vi "HFRR ADV v037 new software.vi"() -> ()   [LabVIEW 2025] (continued)
                    n909 = Number To Fractional String(number=w1103, precision (6)=i16 1) -> (F-format string=w1102:string)  [unwired: 2 in]
                    n910 = local write "Minor Axis"(w1108) -> ()
                    n911 = local write "Major Axis"(w1108) -> ()
                    n912 = Fract/Exp String To Number(string=w1102) -> (number=w1101:dbl)  [unwired: 3 in, 1 out]
                    n913 = local write "Average"(w1101) -> ()
                  }
                }
              }
              frame True {
                w1140 = 1000.0 ("y")
                w1146 = 0.0 ("default (0 DBL)")
                n914 = Match Pattern(string=w1152, regular expression=" \"width_px\":") -> (after substring=w1150:string)  [unwired: 1 in, 3 out]
                n915 = Match Pattern(string=w1150, regular expression="\"height_px\":") -> (before substring=w1148:string, after substring=w1147:string)  [unwired: 1 in, 2 out]
                n916 = Fract/Exp String To Number(string=w1148, default (0 dbl)=w1146) -> (number=w1145:dbl)  [unwired: 2 in, 1 out]
                n917 = Fract/Exp String To Number(string=w1147, default (0 dbl)=w1146) -> (number=w1144:dbl)  [unwired: 2 in, 1 out]
                n918 = Multiply(x=w1145, y=w1143) -> (x*y=w1142:dbl)
                n919 = Multiply(x=w1144, y=w1143) -> (x*y=w1141:dbl)
                n920 = Multiply(x=w1142, y=w1140) -> (x*y=w1126:dbl)
                n921 = Multiply(x=w1141, y=w1140) -> (x*y=w1124:dbl)
                n922 = Add(x=w1126, y=w1124) -> (x+y=w1138:dbl)
                n923 = property on="Major Axis" class="DigNum (strict)"("Caption.Text"="Major Axis") -> ()  [unwired: 2 in, 2 out]
                n924 = property on="Minor Axis" class="DigNum (strict)"("Caption.Text"="Minor Axis") -> ()  [unwired: 2 in, 2 out]
                n925 = property on="Average" class="DigNum (strict)"("Caption.Text"="Average") -> ()  [unwired: 2 in, 2 out]
                n926 = Divide(x=w1138, y=2.0) -> (x/y=w1122:dbl)
                n927 = Bundle By Name(cluster=w1139, "major"=w1126, "minor"=w1124, "average"=w1122) -> (w1136:cluster{"major":dbl, "minor":dbl, "average":dbl})
                n928 = Number To Fractional String(number=w1124, precision (6)=i16 1) -> (F-format string=w1131:string)  [unwired: 2 in]
                n929 = Number To Fractional String(number=w1122, precision (6)=i16 1) -> (F-format string=w1132:string)  [unwired: 2 in]
                n930 = Number To Fractional String(number=w1126, precision (6)=i16 1) -> (F-format string=w1130:string)  [unwired: 2 in]
                n931 = Fract/Exp String To Number(string=w1131) -> (number=w1123:dbl)  [unwired: 3 in, 1 out]
                n932 = Fract/Exp String To Number(string=w1132) -> (number=w1121:dbl)  [unwired: 3 in, 1 out]
                n933 = Fract/Exp String To Number(string=w1130) -> (number=w1125:dbl)  [unwired: 3 in, 1 out]
                n934 = local write "Major Axis"(w1125) -> ()
                n935 = local write "Average"(w1121) -> ()
                n936 = local write "Minor Axis"(w1123) -> ()
              }
            }
            n937 = case shown="\"Measrument\", Default" w1032 {
              tunnel: w1035 -> [w1065 _]
              tunnel: w1034 -> [w1064 _]
              tunnel: [w1061 w1090] -> w1033
              tunnel: w1031 -> [w1063 w1090]
              tunnel: w1030 -> [w1062 _]
              tunnel: w1027 -> [w1060 _]
              frame "Measrument", Default {
                n938 = stacked-sequence {
                  tunnel: w1065 -> [w1083 _]
                  tunnel: w1064 -> [w1081 _]
                  tunnel: w1063 -> [w1079 _]
                  tunnel: w1062 -> [w1078 _]
                  tunnel: [w1073 _] -> w1061
                  tunnel: w1060 -> [w1066 _]
                  frame #0 {
                    n939 = call "IMAGE ANALYSIS.vi"("Enum"=POST_ANALYSIS_ENUM."SAVE IMAGE", "error in"=w1079, "IMAGE FILE PATH"=w1078) -> ("error out"=w1077:errorcluster)  [unwired: 7 in, 1 out]
                    n940 = call "Stall Data Flow.vim"("value in"=w1077, "milliseconds to wait"=u32 1000) -> ("value out"=w1068:errorcluster)  [unwired: 1 out]
                    n941 = local read "Test File List :"() -> (w1085:string)
                    n942 = call "IMAGE ANALYSIS.vi"("Enum"=POST_ANALYSIS_ENUM."MINIMIZE UI", "error in"=w1068) -> ("error out"=w1075:errorcluster)  [unwired: 8 in, 1 out]
                    n943 = Bundle By Name(cluster=T26 {"File Name"="", "Test Method"="", "Operator"="", "Fuel Description"="", "Date and time"=""} ("Main Ref"), "Test Method"=w1066, "File Name"=w1085) -> (w1086:T26)
                    n944 = call "Stall Data Flow.vim"("value in"=w1075, "milliseconds to wait"=u32 1500) -> ("value out"=w1070:errorcluster)  [unwired: 1 out]
                    n945 = call "duf file read.vi"("error in (no error)"=w1070, "Main Ref"=w1086) -> ("error out"=w1084:errorcluster, "Main Ref 2"=w1082:T26)  [unwired: 8 in]
                    n946 = call "DETECTION REPORT for manual.vi"("error in (no error)"=w1084, "return value 3"=w1081, "Image File Path"=w1083, "Main Ref"=w1082) -> ("error out"=w1080:errorcluster)  [unwired: 7 in]
                    n947 = call <vilib>:"Clear Errors.vi"("error in (no error)"=w1080) -> ("error out"=w1071:errorcluster)  [unwired: 5 in, 1 out]
                    n948 = call "IMAGE ANALYSIS.vi"("Enum"=POST_ANALYSIS_ENUM."MINIMIZE UI", "error in"=w1071) -> ("error out"=w1073:errorcluster)  [unwired: 8 in, 1 out]
                  }
                  frame #1 {
                    n949 = local write "Main Tab"(T2."HOME" ("Main Tab")) -> ()
                    n950 = local write "Main Dashboard Buttons"(T1."Home" ("Main Dashboard Buttons")) -> ()
                  }
                }
              }
              frame "Calibrate" {
              }
            }
          }
          frame #2 {
            n951 = Not(x=w1155) -> (.not. x?=w1154:bool)
            n952 = local write "Confirm Measrurement"(w1154) -> ()
            n953 = local read "Calibration Tab"() -> (w1153:enum32{"Measrument", "Calibrate"})
            n954 = case shown="\"Measrument\", Default" w1153 {
              frame "Measrument", Default {
                (unwired) T21."HOME" ("Main Tab")
                n955 = local write "Main Tab"(T2."HOME" ("Main Tab")) -> ()
              }
              frame "Calibrate" {
              }
            }
          }
        }
      }
    }
    n956 = local read "Humidity"() -> (w889:bool)
    n957 = local read "Save Change"() -> (w894:bool)
    n958 = local read "Calibrate"() -> (w895:bool)
    n959 = local read "Auto Start Test"() -> (w890:bool)
    n960 = case shown="True" w895 {
      selector: w895 -> [_ w1002]
      frame False {
      }
      frame True {
        n961 = Not(x=w1002) -> (.not. x?=w1001:bool)
        n962 = local write "Calibrate"(w1001) -> ()
        n963 = local write "Calibration Tab"(enum32{"Measrument", "Calibrate"}."Calibrate" ("Calibration Tab")) -> ()
      }
    }
    n964 = case shown="True" w894 {
      selector: w894 -> [_ w946]
      frame False {
      }
      frame True {
        n965 = stacked-sequence {
          tunnel: w946 -> [_ _ _ _ w1000]
          frame #0 {
            n966 = call "IMAGE ANALYSIS.vi"("Enum"=POST_ANALYSIS_ENUM."HIDE UI") -> ()  [unwired: 9 in, 2 out]
          }
          frame #1 {
            n967 = local read "100x gain"() -> (w948:dbl)
            n968 = local read "10x Gain"() -> (w949:dbl)
            n969 = local read "5x Gain"() -> (w950:dbl)
            n970 = Number To Fractional String(number=w949, width (-)=i16 4, precision (6)=i16 7) -> (F-format string=w971:string)  [unwired: 1 in]
            n971 = Number To Fractional String(number=0.0, width (-)=i16 4, precision (6)=i16 7) -> (F-format string=w966:string)  [unwired: 1 in]
            n972 = Number To Fractional String(number=w948, width (-)=i16 4, precision (6)=i16 7) -> (F-format string=w954:string)  [unwired: 1 in]
            n973 = Number To Fractional String(number=w950, width (-)=i16 10 ("precision (6)"), precision (6)=i16 7) -> (F-format string=w980:string)  [unwired: 1 in]
            n974 = Concatenate Strings("[CH1]" ("string"), w980, " - 5x Gain" ("string"), "\r") -> (w970:string)
            n975 = Concatenate Strings("[CH2]" ("string"), w971, " - 10x Gain" ("string"), "\r") -> (w969:string)
            n976 = Concatenate Strings("[CH3]" ("string"), w966, " - 20x Gain" ("string"), "\r") -> (w960:string)
            n977 = Concatenate Strings("[CH4]" ("string"), w954, " - 100x Gain" ("string"), "\r") -> (w953:string)
            n978 = String To Path(string="C:\\LAB-IQ\\Image Calibrate v01.dcf") -> (path=w983:path)
            n979 = Concatenate Strings(w970, w969, w960, w953) -> (w968:string)
            n980 = call <vilib>:"Write Characters To File.vi"("append to file? (new file:F)"=FALSE, "character string"=w968, "file path (dialog if empty)"=w983) -> ()  [unwired: 2 in, 1 out]
          }
          frame #2 {
            n981 = String To Path(string="C:\\LAB-IQ\\Image Calibrate v01.dcf") -> (path=w986:path)
            n982 = Open/Create/Replace File ("Open File")(file path (use dialog)=w986) -> (refnum out=w987:refnum<file>)  [unwired: 5 in, 2 out]
            n983 = for {
              N: 4 -> [_]
              tunnel: w987 -> [w993]
              i -> [w989]
              n984 = Read from Text File ("Read File")(file (use dialog)=w993) -> (text=w994:string)  [unwired: 3 in, 3 out]
              n985 = String Subset(string=w994, offset (0)=6, length (rest)=10 ("length (rest)")) -> (substring=w990:string)
              n986 = Fract/Exp String To Number(string=w990) -> (number=w988:dbl)  [unwired: 3 in, 1 out]
              n987 = case shown="3" w989 {
                tunnel: w988 -> [w995 w996 _ w997 _]
                frame 0 {
                  n988 = local write "5x Gain"(w995) -> ()
                }
                frame 1 {
                  n989 = local write "10x Gain"(w996) -> ()
                }
                frame 2 {
                }
                frame 3 {
                  n990 = local write "100x gain"(w997) -> ()
                }
                frame 4, Default {
                }
              }
            }
          }
          frame #3 {
            n991 = call "IMAGE ANALYSIS.vi"("Enum"=POST_ANALYSIS_ENUM."SHOW UI") -> ()  [unwired: 9 in, 2 out]
          }
          frame #4 {
            n992 = Not(x=w1000) -> (.not. x?=w999:bool)
            n993 = local write "Save Change"(w999) -> ()
          }
        }
      }
    }
    n994 = case shown="False" w890 {
      tunnel: w889 -> [w916 _]
      frame False {
        n995 = case shown="True" w916 {
          frame False {
          }
          frame True {
            n996 = local read "Set Humidity:"() -> (w920:dbl)
            n997 = local read "Set Humidity:"() -> (w923:dbl)
            n998 = local read "Humidity ( %RH )"() -> (w924:dbl)
            n999 = Subtract(x=w920, y=2.0) -> (x-y=w918:dbl)
            n1000 = Add(x=w923, y=2.0) -> (x+y=w919:dbl)
            n1001 = In Range and Coerce(upper limit=w919, x=w924, lower limit=w918) -> (In Range?=w917:bool)  [unwired: 1 out]
            n1002 = case shown="True" w917 {
              frame False {
              }
              frame True {
                n1003 = case shown="True" "Manual Humididty Reached" {
                  selector: "Manual Humididty Reached" -> [_ w927]
                  frame False {
                  }
                  frame True {
                    n1004 = Not(x=w927) -> (.not. x?=w926:bool)
                    n1005 = local write "Manual Humididty Reached"(w926) -> ()
                    n1006 = local read "EVENT LOG"() -> (w929:string)
                    n1007 = call "Event Log.vi"("Content"="Target Humidity reached", "EVENT LOG"=w929) -> ("EVENT LOG"=w928:string)  [unwired: 8 in, 1 out]
                    n1008 = local write "EVENT LOG"(w928) -> ()
                  }
                }
              }
            }
          }
        }
      }
      frame True {
        n1009 = local write "Manual Humididty Reached"(TRUE ("Manual Humididty Reached")) -> ()
      }
    }
    n1010 = Wait (ms)(milliseconds to wait=u32 250) -> ()  [unwired: 1 out]
    n1011 = local read "Cap Live Image"() -> (w910:bool)
    n1012 = local read "SCAR MEASURMENT"() -> (w913:enum32{"Auto Scar", "Manual Scar"})
    n1013 = Equal?(x=w913, y=enum32{"Auto Scar", "Manual Scar"}."Manual Scar" ("SCAR MEASURMENT")) -> (x = y?=w911:bool)
    n1014 = And(x=w911, y=w910) -> (x .and. y?=w909:bool)
    n1015 = case shown="True" w909 {
      selector: w909 -> [_ w1241]
      frame False {
      }
      frame True {
        n1016 = stacked-sequence {
          tunnel: [_ _ _ w1260 _] -> _
          tunnel: w1241 -> [_ _ _ _ w1267]
          frame #0 {
            w1242 = 0.0
            n1017 = local write "Major Axis"(w1242) -> ()
            n1018 = local write "Minor Axis"(w1242) -> ()
            n1019 = local write "Average"(w1242) -> ()
          }
          frame #1 {
            n1020 = call "CAMERA LIVE FEED FGV.vi"("Enum - Menu"=CAMERA_LIVE_FEED_ENUM."CAMERA MINIMIZE") -> ()  [unwired: 9 in, 2 out]
          }
          frame #2 {
            n1021 = local read "Magnification len live scar"() -> (w1245:string)
            n1022 = case shown="\"10x\", Default" w1245 {
              tunnel: ["_10x" "_5x"] -> w1244
              frame "10x", Default {
              }
              frame "5x" {
              }
            }
            n1023 = local read "FILE 3"() -> (w1252:string)
            n1024 = call <vilib>:"Trim Whitespace.vi"("string"="C:\\LAB-IQ\\images\\") -> ("trimmed string"=w1254:string)  [unwired: 1 in]
            n1025 = String To Path(string=w1254) -> (path=w1253:path)
            n1026 = Concatenate Strings(w1252, w1244, ".png" ("string")) -> (w1251:string)
            n1027 = Build Path(base path=w1253, name or relative path=w1251) -> (appended path=w1250:path)
            n1028 = Path To String(path=w1250) -> (string=w1249:string)
            n1029 = call "CAMERA LIVE FEED FGV.vi"("Enum - Menu"=CAMERA_LIVE_FEED_ENUM."CAMERA SAVE", "Image Path"=w1249) -> ("error out"=w1247:errorcluster)  [unwired: 8 in, 1 out]
            n1030 = case shown="No Error" w1247 {
              frame No Error {
                n1031 = One Button Dialog(message="Image saved successfully") -> ()  [unwired: 1 in, 1 out]
              }
              frame Error {
              }
            }
          }
          frame #3 {
            n1032 = call "LIST FILE NAMES.vi"() -> ("error out"=w1262:errorcluster, "filenames"=w1259:string[])  [unwired: 10 in]
            n1033 = call "IMAGE ANALYSIS.vi"("Enum"=POST_ANALYSIS_ENUM."SHOW UI", "error in"=w1262) -> ("error out"=w1260:errorcluster)  [unwired: 8 in, 1 out]
            n1034 = property on="Test File List :" class="CmbBox"("Strings[]"=w1259) -> ()  [unwired: 2 in, 2 out]
          }
          frame #4 {
            (unwired) T25."Report" ("Main Dashboard Buttons")
            (unwired) T27."Report" ("Main Dashboard Buttons")
            n1035 = Not(x=w1267) -> (.not. x?=w1266:bool)
            n1036 = local write "Zoom Factore"(0.0 ("Zoom Factore")) -> ()
            n1037 = local write "Cap Live Image"(w1266) -> ()
            n1038 = local write "Main Tab"(T2."Adv Scar Report" ("Main Tab")) -> ()
            n1039 = property on="Cap Live Image" class="Bool (strict)"("BoolText.Text"="Capture Image" ("Boolean Text.Text")) -> ()  [unwired: 2 in, 2 out]
            n1040 = local write "Main Dashboard Buttons"(T1."Report" ("Main Dashboard Buttons")) -> ()
          }
        }
      }
    }
    n1041 = local read "change Gain"() -> (w893:bool)
    n1042 = local read "Back Square"() -> (w892:bool)
    n1043 = case shown="True" w893 {
      selector: w893 -> [_ w937]
      frame False {
      }
      frame True {
        n1044 = stacked-sequence {
          tunnel: w937 -> [_ w945]
          frame #0 {
            n1045 = local read "Actual (µm)"() -> (w941:dbl)
            n1046 = local read "Pixel Value"() -> (w940:dbl)
            n1047 = local read "Magnification :"() -> (w939:string)
            n1048 = Divide(x=w941, y=w940) -> (x/y=w938:dbl)
            n1049 = case shown="\"10x\"" w939 {
              tunnel: w938 -> [w942 w943]
              frame "10x" {
                n1050 = local write "10x Gain"(w942) -> ()
              }
              frame "5x", Default {
                n1051 = local write "5x Gain"(w943) -> ()
              }
            }
          }
          frame #1 {
            n1052 = Not(x=w945) -> (.not. x?=w944:bool)
            n1053 = local write "change Gain"(w944) -> ()
          }
        }
      }
    }
    n1054 = case shown="True" w892 {
      selector: w892 -> [_ w935]
      frame False {
      }
      frame True {
        n1055 = Not(x=w935) -> (.not. x?=w934:bool)
        n1056 = local write "Back Square"(w934) -> ()
        n1057 = local write "Calibration Tab"(enum32{"Measrument", "Calibrate"}."Measrument" ("Calibration Tab")) -> ()
      }
    }
    n1058 = local read "Rectangle Tool"() -> (w904:bool)
    n1059 = local read "Clear ROI Tool"() -> (w903:bool)
    n1060 = local read "Open Image"() -> (w908:bool)
    n1061 = local read "line tool"() -> (w905:bool)
    n1062 = local read "OUT"() -> (w906:bool)
    n1063 = local read "In"() -> (w907:bool)
    n1064 = case shown="True" w908 {
      selector: w908 -> [_ w1227]
      tunnel: [w1218 w1229] -> _
      tunnel: w898 -> [w1218 w1228]
      frame False {
      }
      frame True {
        w1220 = "_5x" ("regular expression")
        n1065 = Not(x=w1227) -> (.not. x?=w1226:bool)
        n1066 = local write "Open Image"(w1226) -> ()
        n1067 = call "IMAGE ANALYSIS.vi"("Enum"=POST_ANALYSIS_ENUM."HIDE UI", "error in"=w1228) -> ("error out"=w1236:errorcluster)  [unwired: 8 in, 1 out]
        n1068 = call "File Dialog"("start path"=path "C:/LAB-IQ/images", "error in"=w1236) -> ("selected path"=w1225:path, "error out"=w1234:errorcluster)  [unwired: 10 in, 2 out]
        "Image path  2" <- w1225
        n1069 = call <vilib>:"Clear Errors.vi"("error in (no error)"=w1234) -> ("error out"=w1233:errorcluster)  [unwired: 5 in, 1 out]
        n1070 = call "IMAGE ANALYSIS.vi"("Enum"=POST_ANALYSIS_ENUM."OPEN FILE", "error in"=w1233, "File Path"=w1225) -> ("error out"=w1232:errorcluster)  [unwired: 7 in, 1 out]
        n1071 = call <vilib>:"Clear Errors.vi"("error in (no error)"=w1232) -> ("error out"=w1231:errorcluster)  [unwired: 5 in, 1 out]
        n1072 = call "IMAGE ANALYSIS.vi"("Enum"=POST_ANALYSIS_ENUM."SHOW UI", "error in"=w1231) -> ("error out"=w1229:errorcluster)  [unwired: 8 in, 1 out]
        n1073 = local write "Zoom Factore"(100.0 ("Zoom Factore")) -> ()
        n1074 = local read "Image path  2"() -> (w1221:path)
        n1075 = Strip Path(path=w1221) -> (name=w1223:string)  [unwired: 1 out]
        n1076 = Match Pattern(string=w1223, regular expression=w1220) -> (match substring=w1222:string)  [unwired: 1 in, 3 out]
        n1077 = Equal?(x=w1222, y=w1220) -> (x = y?=w1219:bool)
        n1078 = case shown="True" w1219 {
          frame False {
            n1079 = local write "Magnification :"("10x" ("Magnification :")) -> ()
          }
          frame True {
            n1080 = local write "Magnification :"("5x" ("Magnification :")) -> ()
          }
        }
      }
    }
    n1081 = case shown="True" w906 {
      selector: w906 -> [_ w1203]
      tunnel: w898 -> [w1200 w1208]
      tunnel: [w1200 w1202] -> _
      frame False {
      }
      frame True {
        n1082 = Not(x=w1203) -> (.not. x?=w1201:bool)
        n1083 = local read "Zoom Factore"() -> (w1206:dbl)
        n1084 = local write "OUT"(w1201) -> ()
        n1085 = call "IMAGE ANALYSIS.vi"("Enum"=POST_ANALYSIS_ENUM."ZOOM OUT", "error in"=w1208) -> ("error out"=w1202:errorcluster)  [unwired: 8 in, 1 out]
        n1086 = Divide(x=w1206, y=1.2) -> (x/y=w1204:dbl)
        n1087 = local write "Zoom Factore"(w1204) -> ()
      }
    }
    n1088 = case shown="True" w907 {
      selector: w907 -> [_ w1212]
      tunnel: w898 -> [w1209 w1217]
      tunnel: [w1209 w1210] -> _
      frame False {
      }
      frame True {
        n1089 = Not(x=w1212) -> (.not. x?=w1211:bool)
        n1090 = local read "Zoom Factore"() -> (w1215:dbl)
        n1091 = local write "In"(w1211) -> ()
        n1092 = call "IMAGE ANALYSIS.vi"("Enum"=POST_ANALYSIS_ENUM."ZOOM IN", "error in"=w1217) -> ("error out"=w1210:errorcluster)  [unwired: 8 in, 1 out]
        n1093 = Multiply(x=w1215, y=1.2) -> (x*y=w1213:dbl)
        n1094 = local write "Zoom Factore"(w1213) -> ()
      }
    }
    n1095 = case shown="True" w903 {
      selector: w903 -> [_ w1184]
      tunnel: w898 -> [w1182 w1186]
      tunnel: [w1182 w1185] -> _
      frame False {
      }
      frame True {
        n1096 = Not(x=w1184) -> (.not. x?=w1183:bool)
        n1097 = local write "Clear ROI Tool"(w1183) -> ()
        n1098 = call "IMAGE ANALYSIS.vi"("Enum"=POST_ANALYSIS_ENUM."CLEAR ROI", "error in"=w1186) -> ("error out"=w1185:errorcluster)  [unwired: 8 in, 1 out]
      }
    }
    n1099 = case shown="True" w905 {
      selector: w905 -> [_ w1196]
      tunnel: w898 -> [w1194 w1199]
      tunnel: [w1194 w1197] -> _
      frame False {
      }
      frame True {
        n1100 = Not(x=w1196) -> (.not. x?=w1195:bool)
        n1101 = local write "line tool"(w1195) -> ()
        n1102 = call "IMAGE ANALYSIS.vi"("Enum"=POST_ANALYSIS_ENUM."DRAW LINE", "error in"=w1199) -> ("error out"=w1197:errorcluster)  [unwired: 8 in, 1 out]
      }
    }
    n1103 = case shown="True" w904 {
      selector: w904 -> [_ w1190]
      tunnel: w898 -> [w1188 w1192]
      tunnel: [w1188 w1191] -> _
      frame False {
      }
      frame True {
        n1104 = Not(x=w1190) -> (.not. x?=w1189:bool)
        n1105 = local write "Rectangle Tool"(w1189) -> ()
        n1106 = call "IMAGE ANALYSIS.vi"("Enum"=POST_ANALYSIS_ENUM."DRAW REC", "error in"=w1192) -> ("error out"=w1191:errorcluster)  [unwired: 8 in, 1 out]
      }
    }
    n1107 = local read "SCAR MEASURMENT"() -> (w891:enum32{"Auto Scar", "Manual Scar"})
    n1108 = local read "Fit to Screen Tool"() -> (w900:bool)
    n1109 = local read "Resize Tool"() -> (w899:bool)
    n1110 = case shown="\"Manual Scar\", Default" w891 {
      frame "Auto Scar" {
        n1111 = property on="Cap Live Image" class="Bool (strict)"("BoolText.Text"="Report" ("Boolean Text.Text")) -> ()  [unwired: 2 in, 2 out]
      }
      frame "Manual Scar", Default {
        n1112 = property on="Cap Live Image" class="Bool (strict)"("BoolText.Text"="Save Image" ("Boolean Text.Text")) -> ()  [unwired: 2 in, 2 out]
      }
    }
    n1113 = local read "ROI Color Tool"() -> (w901:bool)
    n1114 = local read "Pan Tool"() -> (w902:bool)
    n1115 = case shown="True" w902 {
      selector: w902 -> [_ w1178]
      tunnel: w898 -> [w1176 w1180]
      tunnel: [w1176 w1179] -> _
      frame False {
      }
      frame True {
        n1116 = Not(x=w1178) -> (.not. x?=w1177:bool)
        n1117 = call "IMAGE ANALYSIS.vi"("Enum"=POST_ANALYSIS_ENUM."PAN", "error in"=w1180) -> ("error out"=w1179:errorcluster)  [unwired: 8 in, 1 out]
        n1118 = local write "Pan Tool"(w1177) -> ()
      }
    }
    n1119 = case shown="True" w899 {
      selector: w899 -> [_ w1162]
      tunnel: w898 -> [w1157 w1159]
      tunnel: [w1157 w1158] -> _
      frame False {
      }
      frame True {
        n1120 = Not(x=w1162) -> (.not. x?=w1161:bool)
        n1121 = local write "Resize Tool"(w1161) -> ()
        n1122 = call "IMAGE ANALYSIS.vi"("Enum"=POST_ANALYSIS_ENUM."RESIZE MODE", "error in"=w1159) -> ("error out"=w1158:errorcluster)  [unwired: 8 in, 1 out]
      }
    }
    n1123 = case shown="True" w900 {
      selector: w900 -> [_ w1167]
      tunnel: [w1163 w1168] -> _
      tunnel: w898 -> [w1163 w1166]
      frame False {
      }
      frame True {
        n1124 = Not(x=w1167) -> (.not. x?=w1165:bool)
        n1125 = local write "Zoom Factore"(100.0 ("Zoom Factore")) -> ()
        n1126 = local write "Fit to Screen Tool"(w1165) -> ()
        n1127 = call "IMAGE ANALYSIS.vi"("Enum"=POST_ANALYSIS_ENUM."FIT", "error in"=w1166) -> ("error out"=w1168:errorcluster)  [unwired: 8 in, 1 out]
      }
    }
    n1128 = case shown="True" w901 {
      selector: w901 -> [_ w1173]
      tunnel: [w1170 w1174] -> _
      tunnel: w898 -> [w1170 w1171]
      frame False {
      }
      frame True {
        n1129 = Not(x=w1173) -> (.not. x?=w1172:bool)
        n1130 = local write "ROI Color Tool"(w1172) -> ()
        n1131 = call "IMAGE ANALYSIS.vi"("Enum"=POST_ANALYSIS_ENUM."SET ROI COLOR", "error in"=w1171) -> ("error out"=w1174:errorcluster)  [unwired: 8 in, 1 out]
      }
    }
    n1132 = local read "Quit"() -> (w915:bool)
  }
  n1133 = while {
    stop <- w1269 stop-if-true
    n1134 = local read "Image Path"() -> (w1272:path)
    n1135 = local read "Print 3"() -> (w1275:bool)
    n1136 = Equal?(x=w1272, y=path "") -> (x = y?=w1271:bool)
    n1137 = Not(x=w1271) -> (.not. x?=w1270:bool)
    n1138 = property on="Print 3" class="Bool (strict)"("Visible"=w1270) -> ()  [unwired: 2 in, 2 out]
    n1139 = case shown="True" w1275 {
      frame False {
        n1140 = local write "Rd"(TRUE ("Boolean 7")) -> ()
      }
      frame True {
        n1141 = flat-sequence {
          tunnel: [w1315] -> w1283
          tunnel: [w1302] -> w1281
          tunnel: [w1312] -> w1277
          tunnel: w1283 -> [w1324]
          tunnel: [w1324] -> w1282
          tunnel: w1281 -> [w1323]
          tunnel: [w1323] -> w1280
          tunnel: [w1321] -> w1279
          tunnel: [w1320] -> w1278
          tunnel: w1277 -> [w1320]
          tunnel: w1282 -> [w1326]
          tunnel: w1280 -> [w1327]
          tunnel: w1279 -> [_]
          tunnel: w1278 -> [w1325]
          frame #0 {
            n1142 = case shown="True" "Rd" {
              frame False {
              }
              frame True {
                n1143 = while {
                  tunnel: "abcdefABCDEF" ("string 2") -> [w1294]
                  shift-right: [w1292] -> w1286
                  shift-left: "" -> [w1291]
                  i -> [w1301]
                  stop <- w1300 stop-if-true
                  n1144 = Random Number (0-1)() -> (number: 0 to 1=w1295:dbl)
                  n1145 = Multiply(x=w1295, y=62.0) -> (x*y=w1297:dbl)
                  n1146 = Decrement(x="Length 2") -> (x-1=w1290:i16)
                  n1147 = To Word Integer(number=w1297) -> (16bit integer=w1298:i16)
                  n1148 = String Subset(string=w1294, offset (0)=w1298, length (rest)=1 ("length (rest)")) -> (substring=w1293:string)
                  n1149 = Greater Or Equal?(x=w1301, y=w1290) -> (x >= y?=w1300:bool)
                  n1150 = Concatenate Strings(w1293, w1291) -> (w1292:string)
                }
                "String 10" <- w1286
                n1151 = local write "Rd"(FALSE ("Boolean 7")) -> ()
              }
            }
          }
          frame #1 {
            w1313 = "_resized.jpg" ("command line")
            (unwired) ".jpg -resize 320x240 " ("string")
            (unwired) "Choose an Image File" ("prompt")
            # "-resize 1798x425"
            n1152 = local read "Image Path"() -> (w1307:path)
            n1153 = Strip Path(path=w1307) -> (stripped path=w1302:path, name=w1303:string)
            n1154 = Match Pattern(string=w1303, regular expression=".jpg") -> (before substring=→"before substring 2":string, after substring=→"after substring":string)  [unwired: 1 in, 2 out]
            n1155 = Match Pattern(string=w1303, regular expression="\\") -> (before substring=w1309:string)  [unwired: 1 in, 3 out]
            n1156 = Match Pattern(string=w1309, regular expression=".jpg") -> (before substring=w1308:string)  [unwired: 1 in, 3 out]
            n1157 = Concatenate Strings("cmd /c convert " ("string"), w1308, ".jpg -resize 320x240  " ("command line"), w1308, w1313) -> (w1316:string)
            n1158 = call <vilib>:"System Exec.vi"("run minimized? (F)"=TRUE, "wait until completion? (T)"=TRUE, "working directory"=w1302, "command line"=w1316) -> ("error out"=w1315:errorcluster)  [unwired: 4 in, 3 out]
            "error out 2" <- w1315
            n1159 = Concatenate Strings(w1308, w1313) -> (w1312:string)
          }
          frame #2 {
            n1160 = Wait (ms)(milliseconds to wait=u32 2000 ("millisecond timer value")) -> (millisecond timer value=w1321:u32)
          }
          frame #3 {
            n1161 = case shown="No Error" w1326 {
              tunnel: w1327 -> [w1330 _]
              tunnel: w1325 -> [w1328 _]
              frame No Error {
                (unwired) ".jpg" ("string")
                n1162 = Path To String(path=w1330) -> (string=w1334:string)
                n1163 = Concatenate Strings(w1334, "\\" ("string"), w1328) -> (w1333:string)
                n1164 = String To Path(string=w1333) -> (path=w1332:path)
                n1165 = call <vilib>:"Read JPEG File.vi"("path to JPEG file"=w1332) -> ("image data"=w1336:T16)  [unwired: 8 in, 2 out]
                "image data" <- w1336
                n1166 = local write "Print 3"(FALSE ("Print 2")) -> ()
                n1167 = call <vilib>:"Draw Flattened Pixmap.vi"("image data"=w1336) -> ("new picture"=→"new picture":picture)  [unwired: 8 in]
              }
              frame Error {
              }
            }
          }
        }
      }
    }
    n1168 = Wait (ms)(milliseconds to wait=u32 20 ("millisecond timer value")) -> ()  [unwired: 1 out]
    n1169 = local read "Quit"() -> (w1269:bool)
  }
  n1170 = while {
    tunnel: w38 -> [_]
    tunnel: w24 -> [_]
    stop <- w1366 stop-if-true
    # "New Adv Logics"
    n1171 = local read "Main Tab"() -> (w1347:T2)
    n1172 = local read "Main Tab"() -> (w1364:T2)
    n1173 = local read "Sign In"() -> (w1363:bool)
    n1174 = case shown="\"Adv Scar\"" w1347 {
      frame "HOME", Default {
        n1175 = local read "LIVE FEED MIN TEMP"() -> (w1499:bool)
        n1176 = local write "LIVE FEED MAX TEMP"(TRUE ("LIVE FEED MAX TEMP")) -> ()
        n1177 = local read "CAMERA ROI MIN TEMP"() -> (w1497:bool)
        n1178 = case shown="True" w1499 {
          selector: w1499 -> [_ w1506]
          frame False {
          }
          frame True {
            n1179 = Not(x=w1506) -> (.not. x?=w1505:bool)
            n1180 = local write "LIVE FEED MIN TEMP"(w1505) -> ()
            n1181 = call "CAMERA LIVE FEED FGV.vi"("Enum - Menu"=CAMERA_LIVE_FEED_ENUM."CAMERA MINIMIZE") -> ()  [unwired: 9 in, 2 out]
          }
        }
        n1182 = case shown="True" w1497 {
          selector: w1497 -> [_ w1503]
          frame False {
          }
          frame True {
            n1183 = Not(x=w1503) -> (.not. x?=w1502:bool)
            n1184 = local write "CAMERA ROI MIN TEMP"(w1502) -> ()
            n1185 = call "IMAGE ANALYSIS.vi"("Enum"=POST_ANALYSIS_ENUM."MINIMIZE UI") -> ()  [unwired: 9 in, 2 out]
          }
        }
        n1186 = local write "CAMERA ROI MAX TEMP"(TRUE ("CAMERA ROI MAX TEMP")) -> ()
      }
      frame "Test Setup" {
        n1187 = local read "LIVE FEED MIN TEMP"() -> (w1509:bool)
        n1188 = local read "CAMERA ROI MIN TEMP"() -> (w1507:bool)
        n1189 = local write "LIVE FEED MAX TEMP"(TRUE ("LIVE FEED MAX TEMP")) -> ()
        n1190 = case shown="True" w1509 {
          selector: w1509 -> [_ w1516]
          frame False {
          }
          frame True {
            n1191 = Not(x=w1516) -> (.not. x?=w1515:bool)
            n1192 = local write "LIVE FEED MIN TEMP"(w1515) -> ()
            n1193 = call "CAMERA LIVE FEED FGV.vi"("Enum - Menu"=CAMERA_LIVE_FEED_ENUM."CAMERA MINIMIZE") -> ()  [unwired: 9 in, 2 out]
          }
        }
        n1194 = case shown="True" w1507 {
          selector: w1507 -> [_ w1513]
          frame False {
          }
          frame True {
            n1195 = Not(x=w1513) -> (.not. x?=w1512:bool)
            n1196 = local write "CAMERA ROI MIN TEMP"(w1512) -> ()
            n1197 = call "IMAGE ANALYSIS.vi"("Enum"=POST_ANALYSIS_ENUM."MINIMIZE UI") -> ()  [unwired: 9 in, 2 out]
          }
        }
        n1198 = local write "CAMERA ROI MAX TEMP"(TRUE ("CAMERA ROI MAX TEMP")) -> ()
      }
      frame "Acquire" {
        n1199 = local read "LIVE FEED MIN TEMP"() -> (w1519:bool)
        n1200 = local write "LIVE FEED MAX TEMP"(TRUE ("LIVE FEED MAX TEMP")) -> ()
        n1201 = local read "CAMERA ROI MIN TEMP"() -> (w1517:bool)
        n1202 = case shown="True" w1519 {
          selector: w1519 -> [_ w1526]
          frame False {
          }
          frame True {
            n1203 = Not(x=w1526) -> (.not. x?=w1525:bool)
            n1204 = local write "LIVE FEED MIN TEMP"(w1525) -> ()
            n1205 = call "CAMERA LIVE FEED FGV.vi"("Enum - Menu"=CAMERA_LIVE_FEED_ENUM."CAMERA MINIMIZE") -> ()  [unwired: 9 in, 2 out]
          }
        }
        n1206 = case shown="True" w1517 {
          selector: w1517 -> [_ w1523]
          frame False {
          }
          frame True {
            n1207 = Not(x=w1523) -> (.not. x?=w1522:bool)
            n1208 = local write "CAMERA ROI MIN TEMP"(w1522) -> ()
            n1209 = call "IMAGE ANALYSIS.vi"("Enum"=POST_ANALYSIS_ENUM."MINIMIZE UI") -> ()  [unwired: 9 in, 2 out]
          }
        }
        n1210 = local write "CAMERA ROI MAX TEMP"(TRUE ("CAMERA ROI MAX TEMP")) -> ()
      }
      frame "Adv Scar" {
        n1211 = local read "CAMERA ROI MIN TEMP"() -> (w1527:bool)
        n1212 = case shown="True" "LIVE FEED MAX TEMP" {
          selector: "LIVE FEED MAX TEMP" -> [_ w1548]
          frame False {
          }
          frame True {
            n1213 = Not(x=w1548) -> (.not. x?=w1547:bool)
            n1214 = local write "LIVE FEED MAX TEMP"(w1547) -> ()
            n1215 = call "CAMERA LIVE FEED FGV.vi"("Enum - Menu"=CAMERA_LIVE_FEED_ENUM."CAMERA RESTORE") -> ("error out"=w1538:errorcluster)  [unwired: 9 in, 1 out]
            n1216 = Type Cast(type=30, x=0) -> (*(type *) &x=w1542:i32)
            n1217 = Add(x=w1542, y=48) -> (x+y=w1543:i32)
            n1218 = call "CAMERA LIVE FEED FGV.vi"("Enum - Menu"=CAMERA_LIVE_FEED_ENUM."CAMERA MODE SET", "error in (no error)"=w1538, "CAMERA MODE"=w1543) -> ("error out"=w1535:errorcluster)  [unwired: 7 in, 1 out]
            n1219 = call "CAMERA LIVE FEED FGV.vi"("Enum - Menu"=CAMERA_LIVE_FEED_ENUM."CAMERA GRAY", "error in (no error)"=w1535) -> ("error out"=w1534:errorcluster)  [unwired: 8 in, 1 out]
            n1220 = call "LIST FILE NAMES.vi"("error in (no error)"=w1534) -> ("error out"=w1544:errorcluster, "filenames"=w1545:string[])  [unwired: 9 in]
            n1221 = property on="FILE 3" class="CmbBox"(error in=w1544, "Strings[]"=w1545) -> ()  [unwired: 1 in, 2 out]
          }
        }
        n1222 = case shown="True" w1527 {
          selector: w1527 -> [_ w1533]
          frame False {
          }
          frame True {
            n1223 = Not(x=w1533) -> (.not. x?=w1532:bool)
            n1224 = local write "CAMERA ROI MIN TEMP"(w1532) -> ()
            n1225 = call "IMAGE ANALYSIS.vi"("Enum"=POST_ANALYSIS_ENUM."MINIMIZE UI") -> ()  [unwired: 9 in, 2 out]
          }
        }
        n1226 = local write "CAMERA ROI MAX TEMP"(TRUE ("CAMERA ROI MAX TEMP")) -> ()
        "LIVE FEED MIN TEMP" <- TRUE ("LIVE FEED MIN TEMP")
      }
      frame "Adv Scar Report" {
        n1227 = local read "CAMERA ROI MAX TEMP"() -> (w1549:bool)
        n1228 = local read "LIVE FEED MIN TEMP"() -> (w1551:bool)
        n1229 = local write "LIVE FEED MAX TEMP"(TRUE ("LIVE FEED MAX TEMP")) -> ()
        n1230 = case shown="True" w1551 {
          selector: w1551 -> [_ w1560]
          frame False {
          }
          frame True {
            n1231 = Not(x=w1560) -> (.not. x?=w1559:bool)
            n1232 = local write "LIVE FEED MIN TEMP"(w1559) -> ()
            n1233 = call "CAMERA LIVE FEED FGV.vi"("Enum - Menu"=CAMERA_LIVE_FEED_ENUM."CAMERA MINIMIZE") -> ()  [unwired: 9 in, 2 out]
          }
        }
        n1234 = case shown="True" w1549 {
          selector: w1549 -> [_ w1557]
          frame False {
          }
          frame True {
            n1235 = Not(x=w1557) -> (.not. x?=w1555:bool)
            n1236 = local write "CAMERA ROI MAX TEMP"(w1555) -> ()
            n1237 = call "IMAGE ANALYSIS.vi"("Enum"=POST_ANALYSIS_ENUM."SHOW UI") -> ("error out"=w1554:errorcluster)  [unwired: 9 in, 1 out]
            n1238 = call "LIST FILE NAMES.vi"("error in (no error)"=w1554) -> ("filenames"=w1553:string[])  [unwired: 9 in, 1 out]
            n1239 = property on="Test File List :" class="CmbBox"("Strings[]"=w1553) -> ()  [unwired: 2 in, 2 out]
          }
        }
        n1240 = local write "CAMERA ROI MIN TEMP"(TRUE ("CAMERA ROI MIN TEMP")) -> ()
      }
      frame "Compare Files" {
        n1241 = local read "LIVE FEED MIN TEMP"() -> (w1563:bool)
        n1242 = local write "LIVE FEED MAX TEMP"(TRUE ("LIVE FEED MAX TEMP")) -> ()
        n1243 = local read "CAMERA ROI MIN TEMP"() -> (w1561:bool)
        n1244 = case shown="True" w1563 {
          selector: w1563 -> [_ w1570]
          frame False {
          }
          frame True {
            n1245 = Not(x=w1570) -> (.not. x?=w1569:bool)
            n1246 = local write "LIVE FEED MIN TEMP"(w1569) -> ()
            n1247 = call "CAMERA LIVE FEED FGV.vi"("Enum - Menu"=CAMERA_LIVE_FEED_ENUM."CAMERA MINIMIZE") -> ()  [unwired: 9 in, 2 out]
          }
        }
        n1248 = case shown="True" w1561 {
          selector: w1561 -> [_ w1567]
          frame False {
          }
          frame True {
            n1249 = Not(x=w1567) -> (.not. x?=w1566:bool)
            n1250 = local write "CAMERA ROI MIN TEMP"(w1566) -> ()
            n1251 = call "IMAGE ANALYSIS.vi"("Enum"=POST_ANALYSIS_ENUM."MINIMIZE UI") -> ()  [unwired: 9 in, 2 out]
          }
        }
        n1252 = local write "CAMERA ROI MAX TEMP"(TRUE ("CAMERA ROI MAX TEMP")) -> ()
      }
      frame "About" {
        n1253 = local read "LIVE FEED MIN TEMP"() -> (w1573:bool)
        n1254 = local write "LIVE FEED MAX TEMP"(TRUE ("LIVE FEED MAX TEMP")) -> ()
        n1255 = local read "CAMERA ROI MIN TEMP"() -> (w1572:bool)
        n1256 = case shown="True" w1573 {
          selector: w1573 -> [_ w1580]
          frame False {
          }
          frame True {
            n1257 = Not(x=w1580) -> (.not. x?=w1579:bool)
            n1258 = local write "LIVE FEED MIN TEMP"(w1579) -> ()
            n1259 = call "CAMERA LIVE FEED FGV.vi"("Enum - Menu"=CAMERA_LIVE_FEED_ENUM."CAMERA MINIMIZE") -> ()  [unwired: 9 in, 2 out]
          }
        }
        n1260 = case shown="True" w1572 {
          selector: w1572 -> [_ w1577]
          frame False {
          }
          frame True {
            n1261 = Not(x=w1577) -> (.not. x?=w1576:bool)
            n1262 = local write "CAMERA ROI MIN TEMP"(w1576) -> ()
            n1263 = call "IMAGE ANALYSIS.vi"("Enum"=POST_ANALYSIS_ENUM."MINIMIZE UI") -> ()  [unwired: 9 in, 2 out]
          }
        }
        n1264 = local write "CAMERA ROI MAX TEMP"(TRUE ("CAMERA ROI MIN TEMP")) -> ()
      }
      frame "Advance" {
        n1265 = local read "LIVE FEED MIN TEMP"() -> (w1583:bool)
        n1266 = local write "LIVE FEED MAX TEMP"(TRUE ("LIVE FEED MAX TEMP")) -> ()
        n1267 = local read "CAMERA ROI MIN TEMP"() -> (w1581:bool)
        n1268 = case shown="True" w1583 {
          selector: w1583 -> [_ w1590]
          frame False {
          }
          frame True {
            n1269 = Not(x=w1590) -> (.not. x?=w1589:bool)
            n1270 = local write "LIVE FEED MIN TEMP"(w1589) -> ()
            n1271 = call "CAMERA LIVE FEED FGV.vi"("Enum - Menu"=CAMERA_LIVE_FEED_ENUM."CAMERA MINIMIZE") -> ()  [unwired: 9 in, 2 out]
          }
        }
        n1272 = local write "CAMERA ROI MAX TEMP"(TRUE ("CAMERA ROI MAX TEMP")) -> ()
        n1273 = case shown="True" w1581 {
          selector: w1581 -> [_ w1587]
          frame False {
          }
          frame True {
            n1274 = Not(x=w1587) -> (.not. x?=w1586:bool)
            n1275 = local write "CAMERA ROI MIN TEMP"(w1586) -> ()
            n1276 = call "IMAGE ANALYSIS.vi"("Enum"=POST_ANALYSIS_ENUM."MINIMIZE UI") -> ()  [unwired: 9 in, 2 out]
          }
        }
      }
      frame "Mooha" {
        n1277 = local read "LIVE FEED MIN TEMP"() -> (w1593:bool)
        n1278 = local write "LIVE FEED MAX TEMP"(TRUE ("LIVE FEED MAX TEMP")) -> ()
        n1279 = local read "CAMERA ROI MIN TEMP"() -> (w1591:bool)
        n1280 = case shown="True" w1593 {
          selector: w1593 -> [_ w1600]
          frame False {
          }
          frame True {
            n1281 = Not(x=w1600) -> (.not. x?=w1599:bool)
            n1282 = local write "LIVE FEED MIN TEMP"(w1599) -> ()
            n1283 = call "CAMERA LIVE FEED FGV.vi"("Enum - Menu"=CAMERA_LIVE_FEED_ENUM."CAMERA MINIMIZE") -> ()  [unwired: 9 in, 2 out]
          }
        }
        n1284 = local write "CAMERA ROI MAX TEMP"(TRUE ("CAMERA ROI MAX TEMP")) -> ()
        n1285 = case shown="True" w1591 {
          selector: w1591 -> [_ w1597]
          frame False {
          }
          frame True {
            n1286 = Not(x=w1597) -> (.not. x?=w1596:bool)
            n1287 = local write "CAMERA ROI MIN TEMP"(w1596) -> ()
            n1288 = call "IMAGE ANALYSIS.vi"("Enum"=POST_ANALYSIS_ENUM."MINIMIZE UI") -> ()  [unwired: 9 in, 2 out]
          }
        }
      }
    }
    n1289 = local read "Auto Start Test"() -> (w1338:bool)
    n1290 = case shown="True" "sign in temp" {
      frame False {
      }
      frame True {
        w1373 = 1 ("y")
        n1291 = local read "USERNAME"() -> (w1379:string)
        n1292 = local read "USER ID"() -> (w1376:string)
        n1293 = call <vilib>:"Trim Whitespace.vi"("string"=w1379) -> ("trimmed string"=w1378:string)  [unwired: 1 in]
        n1294 = call <vilib>:"Trim Whitespace.vi"("string"=w1376) -> ("trimmed string"=w1377:string)  [unwired: 1 in]
        n1295 = String Length(string=w1378) -> (length=w1375:i32)
        n1296 = String Length(string=w1377) -> (length=w1374:i32)
        n1297 = Greater?(x=w1375, y=w1373) -> (0:w1372:bool)
        n1298 = Greater?(x=w1374, y=w1373) -> (0:w1371:bool)
        n1299 = And(x=w1372, y=w1371) -> (x .and. y?=w1370:bool)
        n1300 = case shown="True" w1370 {
          frame False {
            n1301 = property on="Sign In" class="Bool (strict)"("DisabledEnum"=T19."Disabled" ("Disabled")) -> ()  [unwired: 2 in, 2 out]
          }
          frame True {
            n1302 = property on="Sign In" class="Bool (strict)"("DisabledEnum"=T19."Enabled" ("Disabled")) -> ()  [unwired: 2 in, 2 out]
          }
        }
      }
    }
    n1303 = local read "Air Temperature"() -> (w1355:bool)
    n1304 = local read "Coefficient Of Friction"() -> (w1356:bool)
    n1305 = case shown="False" w1338 {
      frame False {
        n1306 = local read "Auto stop temp"() -> (w1367:bool)
        n1307 = case shown="True" w1367 {
          frame False {
          }
          frame True {
            n1308 = local write "Auto Start Temp"(FALSE ("Auto Start Temp")) -> ()
          }
        }
      }
      frame True {
        "Auto stop temp" <- TRUE ("Auto stop temp")
      }
    }
    n1309 = local read "Humidity 2"() -> (w1354:bool)
    n1310 = case shown="\"HOME\"" w1364 {
      frame "HOME" {
        n1311 = local write "main tab sub"(enum32{"Page 1", "Page 2"}."Page 1" ("main tab sub")) -> ()
      }
      frame Default {
        n1312 = local write "main tab sub"(enum32{"Page 1", "Page 2"}."Page 2" ("main tab sub")) -> ()
      }
    }
    n1313 = case shown="True" w1363 {
      selector: w1363 -> [_ w1715]
      frame False {
      }
      frame True {
        n1314 = Not(x=w1715) -> (.not. x?=w1714:bool)
        n1315 = local write "Sign In"(w1714) -> ()
        n1316 = local write "Main Dashboard Buttons"(T25."Test Setup" ("Main Dashboard Buttons")) -> ()
      }
    }
    n1317 = case shown="\"Numeric Display\", Default" "Num/Graph" {
      frame "Numeric Display", Default {
        n1318 = property on="Single/Multiple" class="RadioBtnsControl (strict)"("Visible"=FALSE) -> ()  [unwired: 2 in, 2 out]
        n1319 = property on="Single - Graph" class="Ring (strict)"("Visible"=FALSE) -> ()  [unwired: 2 in, 2 out]
        n1320 = local write "Main Tab Display"(T4."Dashboard 1" ("Main Tab Display")) -> ()
      }
      frame "Graph Display" {
        n1321 = property on="Single/Multiple" class="RadioBtnsControl (strict)"("Visible"=TRUE) -> ()  [unwired: 2 in, 2 out]
        n1322 = case shown="\"Multiple\"" "Single/Multiple" {
          frame "Single ", Default {
            n1323 = property on="Single - Graph" class="Ring (strict)"("Visible"=TRUE) -> ()  [unwired: 2 in, 2 out]
            n1324 = local write "Main Tab Display"(T4."Dashboard 3" ("Main Tab Display")) -> ()
          }
          frame "Multiple" {
            n1325 = property on="Single - Graph" class="Ring (strict)"("Visible"=FALSE) -> ()  [unwired: 2 in, 2 out]
            n1326 = local write "Main Tab Display"(T4."Dashboard 2" ("Main Tab Display")) -> ()
          }
        }
      }
    }
    n1327 = local read "Stroke"() -> (w1353:bool)
    n1328 = local read "USERNAME"() -> (w1358:string)
    n1329 = case shown="True" w1356 {
      selector: w1356 -> [_ w1640]
      frame False {
      }
      frame True {
        n1330 = Not(x=w1640) -> (.not. x?=w1639:bool)
        n1331 = local write "Coefficient Of Friction"(w1639) -> ()
        n1332 = local write "Tab Control 2"(T6."Coefficient Of Friction" ("Tab Control 2")) -> ()
      }
    }
    n1333 = case shown="True" w1355 {
      selector: w1355 -> [_ w1637]
      frame False {
      }
      frame True {
        n1334 = Not(x=w1637) -> (.not. x?=w1635:bool)
        n1335 = local write "Air Temperature"(w1635) -> ()
        n1336 = local write "Tab Control 2"(T6."Air Temperature" ("Tab Control 2")) -> ()
      }
    }
    n1337 = case shown="True" w1353 {
      selector: w1353 -> [_ w1631]
      frame False {
      }
      frame True {
        n1338 = Not(x=w1631) -> (.not. x?=w1629:bool)
        n1339 = local write "Stroke"(w1629) -> ()
        n1340 = local write "Tab Control 2"(T6."Stroke" ("Tab Control 2")) -> ()
      }
    }
    n1341 = local write "tested by"(w1358) -> ()
    n1342 = case shown="True" w1354 {
      selector: w1354 -> [_ w1634]
      frame False {
      }
      frame True {
        n1343 = Not(x=w1634) -> (.not. x?=w1632:bool)
        n1344 = local write "Humidity 2"(w1632) -> ()
        n1345 = local write "Tab Control 2"(T6."Humidity" ("Tab Control 2")) -> ()
      }
    }
    n1346 = case shown="\"Calibration\"" "Main Dashboard Buttons" {
      tunnel: [T2."HOME" ("Main Tab") T2."Test Setup" ("Main Tab") T2."Acquire" ("Main Tab") T2."Adv Scar" ("Main Tab") T2."Adv Scar Report" ("Main Tab") T2."Compare Files" ("Main Tab") T2."Calibration" ("Main Tab") T2."About" ("Main Tab") T2."Advance" ("Main Tab")] -> w1337
      frame "Home", Default {
      }
      frame "Test Setup" {
      }
      frame "Dashboard" {
      }
      frame "Imaging" {
      }
      frame "Report" {
      }
      frame "Analysis" {
      }
      frame "Calibration" {
      }
      frame "About" {
      }
      frame "Advance" {
      }
    }
    n1347 = Wait (ms)(milliseconds to wait=u32 100) -> ()  [unwired: 1 out]
    n1348 = local read "Main Tab Display"() -> (w1357:T4)
    n1349 = local write "Main Tab"(w1337) -> ()
    n1350 = case shown="\"Dashboard 3\"" w1357 {
      frame "Dashboard 1", Default {
        n1351 = property on="Reset Graph" class="Bool (strict)"("Visible"=FALSE) -> ()  [unwired: 2 in, 2 out]
      }
      frame "Dashboard 2" {
        n1352 = property on="Reset Graph" class="Bool (strict)"("Visible"=TRUE) -> ()  [unwired: 2 in, 2 out]
      }
      frame "Dashboard 3" {
        n1353 = property on="Reset Graph" class="Bool (strict)"("Visible"=TRUE) -> ()  [unwired: 2 in, 2 out]
      }
    }
    n1354 = local read "SCAR MEASURMENT"() -> (w1345:enum32{"Auto Scar", "Manual Scar"})
    n1355 = local read "Humidity"() -> (w1359:bool)
    n1356 = local read "Cap Live Image"() -> (w1342:bool)
    n1357 = local read "Sample Temperature"() -> (w1352:bool)
    n1358 = local read "Air Temp vs Humidity"() -> (w1350:bool)
    n1359 = local read "Frequency"() -> (w1351:bool)
    n1360 = case shown="True" w1359 {
      frame False {
        n1361 = local write "Humidity On Command"(TRUE ("Humidity On Command")) -> ()
        n1362 = case shown="True" "Humidity Off Command" {
          selector: "Humidity Off Command" -> [_ w1647]
          frame False {
          }
          frame True {
            n1363 = stacked-sequence {
              frame #0 {
                n1364 = Wait (ms)(milliseconds to wait=u32 500) -> ()  [unwired: 1 out]
              }
              frame #1 {
                n1365 = local read "WriteHumidity"() -> (w1650:string[])
                n1366 = Insert Into Array(array=w1650, new element="R;1" ("new element/subarray")) -> (w1649:string[])  [unwired: 1 in]
                n1367 = local write "WriteHumidity"(w1649) -> ()
              }
              frame #2 {
                n1368 = Wait (ms)(milliseconds to wait=u32 500) -> ()  [unwired: 1 out]
              }
              frame #3 {
                n1369 = local read "WriteHumidity"() -> (w1653:string[])
                n1370 = local read "EVENT LOG"() -> (w1657:string)
                n1371 = call "Event Log.vi"("Content"="Humidity Control Off" ("string"), "EVENT LOG"=w1657) -> ("EVENT LOG"=w1658:string)  [unwired: 8 in, 1 out]
                n1372 = local write "EVENT LOG"(w1658) -> ()
                n1373 = Insert Into Array(array=w1653, new element="R;1" ("new element/subarray")) -> (w1654:string[])  [unwired: 1 in]
                n1374 = local write "WriteHumidity"(w1654) -> ()
              }
            }
            n1375 = Not(x=w1647) -> (.not. x?=w1646:bool)
            n1376 = local write "Humidity Off Command"(w1646) -> ()
          }
        }
      }
      frame True {
        n1377 = local write "Humidity Off Command"(TRUE ("Humidity Off Command")) -> ()
        n1378 = case shown="True" "Humidity On Command" {
          selector: "Humidity On Command" -> [_ w1662]
          frame False {
          }
          frame True {
            n1379 = stacked-sequence {
              frame #0 {
                n1380 = local read "Set Rh"() -> (w1668:dbl)
                n1381 = local read "WriteHumidity"() -> (w1664:string[])
                n1382 = Number To Fractional String(number=w1668, precision (6)=i16 2) -> (F-format string=w1669:string)  [unwired: 2 in]
                n1383 = Concatenate Strings("M;" ("new element/subarray"), w1669) -> (w1667:string)
                n1384 = Insert Into Array(array=w1664, new element=w1667) -> (w1663:string[])  [unwired: 1 in]
                n1385 = local write "WriteHumidity"(w1663) -> ()
              }
              frame #1 {
                n1386 = Wait (ms)(milliseconds to wait=u32 500) -> ()  [unwired: 1 out]
              }
              frame #2 {
                n1387 = local read "WriteHumidity"() -> (w1672:string[])
                n1388 = local read "Set Rh"() -> (w1676:dbl)
                n1389 = Number To Fractional String(number=w1676, precision (6)=i16 2) -> (F-format string=w1677:string)  [unwired: 2 in]
                n1390 = Concatenate Strings("M;" ("new element/subarray"), w1677) -> (w1675:string)
                n1391 = Insert Into Array(array=w1672, new element=w1675) -> (w1671:string[])  [unwired: 1 in]
                n1392 = local write "WriteHumidity"(w1671) -> ()
              }
              frame #3 {
                n1393 = Wait (ms)(milliseconds to wait=u32 500) -> ()  [unwired: 1 out]
              }
              frame #4 {
                (unwired) "% RH" ("string")
                (unwired) i16 2 ("precision (6)")
                (unwired) "M;" ("new element/subarray")
                n1394 = local read "Set Rh"() -> (w1686:dbl)
                n1395 = local read "WriteHumidity"() -> (w1679:string[])
                n1396 = Number To Fractional String(number=w1686, precision (6)=i16 2) -> (F-format string=w1683:string)  [unwired: 2 in]
                n1397 = Concatenate Strings("M;" ("new element/subarray"), w1683) -> (w1687:string)
                n1398 = Concatenate Strings("Humidity Set to : " ("string"), w1683, "% RH" ("string")) -> (w1681:string)
                n1399 = Insert Into Array(array=w1679, new element=w1687) -> (w1680:string[])  [unwired: 1 in]
                n1400 = disable-structure shown="Enabled" {
                  frame Enabled {
                    n1401 = local read "EVENT LOG"() -> (w1690:string)
                    n1402 = call "Event Log.vi"("Content"="Humidity Control On", "EVENT LOG"=w1690) -> ("EVENT LOG"=w1691:string)  [unwired: 8 in, 1 out]
                    n1403 = local write "EVENT LOG"(w1691) -> ()
                  }
                  frame Disabled {
                  }
                }
                n1404 = disable-structure shown="Enabled" {
                  disable-tunnel: w1681 -> [_ _]
                  frame Enabled {
                    n1405 = local read "EVENT LOG"() -> (w1693:string)
                    n1406 = call "Event Log.vi"("Content"="Humidity Control On", "EVENT LOG"=w1693) -> ("EVENT LOG"=w1694:string)  [unwired: 8 in, 1 out]
                    n1407 = local write "EVENT LOG"(w1694) -> ()
                  }
                  frame Disabled {
                  }
                }
                n1408 = local write "WriteHumidity"(w1680) -> ()
              }
            }
            n1409 = Not(x=w1662) -> (.not. x?=w1661:bool)
            n1410 = local write "Humidity On Command"(w1661) -> ()
          }
        }
      }
    }
    n1411 = Equal?(x=w1345, y=enum32{"Auto Scar", "Manual Scar"}."Auto Scar" ("SCAR MEASURMENT")) -> (x = y?=w1341:bool)
    n1412 = local read "TEST STANDARD"() -> (w1348:T3)
    n1413 = And(x=w1342, y=w1341) -> (x .and. y?=w1343:bool)
    n1414 = case shown="True" w1343 {
      selector: w1343 -> [_ w1446]
      tunnel: errorcluster {"status"=FALSE, "code"=0, "source"=""} ("error in (no error) 3") -> [_ w1447]
      frame False {
      }
      frame True {
        n1415 = stacked-sequence {
          tunnel: w1447 -> [_ _ _ _ _ _ _ w1495]
          tunnel: w1446 -> [_ _ _ _ _ w1476 _ _]
          frame #0 {
            n1416 = call "CAMERA LIVE FEED FGV.vi"("Enum - Menu"=CAMERA_LIVE_FEED_ENUM."CAMERA MINIMIZE") -> ()  [unwired: 9 in, 2 out]
          }
          frame #1 {
            n1417 = property on="Auto Scar Check  2" class="Clust (strict)"("Visible"=TRUE) -> ()  [unwired: 2 in, 2 out]
          }
          frame #2 {
            n1418 = String To Path(string="C:\\LAB-IQ\\Image Calibrate v01.dcf") -> (path=w1452:path)
            n1419 = Open/Create/Replace File ("Open File")(file path (use dialog)=w1452) -> (refnum out=w1453:refnum<file>)  [unwired: 5 in, 2 out]
            n1420 = for {
              N: 4 -> [_]
              tunnel: w1453 -> [w1459]
              i -> [w1455]
              n1421 = Read from Text File ("Read File")(file (use dialog)=w1459) -> (text=w1460:string)  [unwired: 3 in, 3 out]
              n1422 = String Subset(string=w1460, offset (0)=6, length (rest)=10 ("length (rest)")) -> (substring=w1456:string)
              n1423 = Fract/Exp String To Number(string=w1456) -> (number=w1454:dbl)  [unwired: 3 in, 1 out]
              n1424 = case shown="0" w1455 {
                tunnel: w1454 -> [w1461 w1462 _ w1463 _]
                frame 0 {
                  "5x Gain" <- w1461
                }
                frame 1 {
                  "10x Gain" <- w1462
                }
                frame 2 {
                }
                frame 3 {
                  "100x gain" <- w1463
                }
                frame 4, Default {
                }
              }
            }
          }
          frame #3 {
            n1425 = local read "FILE 3"() -> (w1469:string)
            n1426 = call <vilib>:"Trim Whitespace.vi"("string"="C:\\LAB-IQ\\images\\") -> ("trimmed string"=w1471:string)  [unwired: 1 in]
            n1427 = String To Path(string=w1471) -> (path=w1470:path)
            n1428 = Concatenate Strings(w1469, ".png" ("string")) -> (w1468:string)
            n1429 = Build Path(base path=w1470, name or relative path=w1468) -> (appended path=w1466:path)
            "Image path" <- w1466
            n1430 = Path To String(path=w1466) -> (string=w1465:string)
            n1431 = call "CAMERA LIVE FEED FGV.vi"("Enum - Menu"=CAMERA_LIVE_FEED_ENUM."CAMERA SAVE", "Image Path"=w1465) -> ()  [unwired: 8 in, 2 out]
          }
          frame #4 {
            n1432 = One Button Dialog(message="Image saved successfully") -> ()  [unwired: 1 in, 1 out]
          }
          frame #5 {
            n1433 = local read "TEST STANDARD"() -> (w1475:T3)
            n1434 = local read "Magnification len live scar"() -> (w1487:string)
            n1435 = Not(x=w1476) -> (.not. x?=w1477:bool)
            n1436 = local write "Cap Live Image"(w1477) -> ()
            n1437 = case shown="\"ISO 12156\"" w1475 {
              tunnel: ["ASTM D6079" "ISO 12156"] -> w1474
              frame "ASTM D6079", Default {
              }
              frame "ISO 12156" {
              }
            }
            n1438 = case shown="\"5x\", Default" w1487 {
              tunnel: [w1490 w1491] -> w1486
              frame "5x", Default {
                n1439 = local read "5x Gain"() -> (w1490:dbl)
              }
              frame "10x" {
                # "5x"
                n1440 = local read "10x Gain"() -> (w1491:dbl)
              }
            }
            n1441 = local read "Image path"() -> (w1485:path)
            n1442 = local read "FILE 3"() -> (w1478:string)
            n1443 = call "EDGE DETCTION.vi"("GAIN VALUE"=w1486, "Image Path"=w1485) -> ("error out"=w1484:errorcluster, "return value"=w1483:cluster{string, string, dbl, dbl, dbl})  [unwired: 8 in]
            n1444 = Bundle By Name(cluster=T26 {"File Name"="", "Test Method"="", "Operator"="", "Fuel Description"="", "Date and time"=""} ("Main Ref"), "File Name"=w1478, "Test Method"=w1474) -> (w1479:T26)
            n1445 = call "duf file read.vi"("error in (no error)"=w1484, "Main Ref"=w1479) -> ("error out"=w1482:errorcluster, "Main Ref 2"=w1480:T26)  [unwired: 8 in]
            n1446 = call "EDGE DETECTION REPORT.vi"("error in (no error)"=w1482, "return value 2"=w1483, "Main Ref"=w1480) -> ()  [unwired: 8 in, 1 out]
          }
          frame #6 {
            n1447 = property on="Auto Scar Check  2" class="Clust (strict)"("Visible"=FALSE) -> ()  [unwired: 2 in, 2 out]
          }
          frame #7 {
            n1448 = call "CAMERA LIVE FEED FGV.vi"("Enum - Menu"=CAMERA_LIVE_FEED_ENUM."CAMERA MINIMIZE", "error in (no error)"=w1495) -> ()  [unwired: 8 in, 2 out]
            n1449 = local write "Main Dashboard Buttons"(T1."Home" ("Main Dashboard Buttons")) -> ()
            n1450 = local write "Main Tab"(T2."HOME" ("Main Tab")) -> ()
          }
        }
      }
    }
    n1451 = local read "Heater Button"() -> (w1349:bool)
    n1452 = case shown="True" w1351 {
      selector: w1351 -> [_ w1625]
      frame False {
      }
      frame True {
        n1453 = Not(x=w1625) -> (.not. x?=w1623:bool)
        n1454 = local write "Frequency"(w1623) -> ()
        n1455 = local write "Tab Control 2"(T6."Frequency" ("Tab Control 2")) -> ()
      }
    }
    n1456 = case shown="True" w1350 {
      selector: w1350 -> [_ w1622]
      frame False {
      }
      frame True {
        n1457 = Not(x=w1622) -> (.not. x?=w1620:bool)
        n1458 = local write "Air Temp vs Humidity"(w1620) -> ()
        n1459 = local write "Tab Control 2"(T6."Air Temp vs Rh" ("Tab Control 2")) -> ()
      }
    }
    n1460 = case shown="True" w1352 {
      selector: w1352 -> [_ w1628]
      frame False {
      }
      frame True {
        n1461 = Not(x=w1628) -> (.not. x?=w1626:bool)
        n1462 = local write "Sample Temperature"(w1626) -> ()
        n1463 = local write "Tab Control 2"(T6."Sample Temperature" ("Tab Control 2")) -> ()
      }
    }
    n1464 = case shown="\"Custom\"" w1348 {
      frame "ASTM D6079", Default {
        w1601 = "ASTM D6079 TEST CONDITIONS" ("Standard 2")
        n1465 = local write "Standard 2"(w1601) -> ()
        n1466 = local write "Standard"(w1601) -> ()
      }
      frame "ISO 12156" {
        w1602 = "ISO 12156 TEST CONDITIONS" ("Standard 2")
        n1467 = local write "Standard 2"(w1602) -> ()
        n1468 = local write "Standard"(w1602) -> ()
      }
      frame "CEC F-096-A-06" {
        w1603 = "CEC F-096-A-06 TEST CONDITIONS" ("Standard 2")
        n1469 = local write "Standard 2"(w1603) -> ()
        n1470 = local write "Standard"(w1603) -> ()
      }
      frame "Custom" {
        w1604 = "CUSTOM TEST CONDITIONS" ("Standard 2")
        n1471 = local write "Standard 2"(w1604) -> ()
        n1472 = local write "Standard"(w1604) -> ()
      }
    }
    n1473 = case shown="True" w1349 {
      frame False {
        n1474 = local write "Temperature On Command"(TRUE ("Temperature On Command")) -> ()
        n1475 = case shown="True" "Temperature Off Command" {
          selector: "Temperature Off Command" -> [_ w1608]
          frame False {
          }
          frame True {
            n1476 = Not(x=w1608) -> (.not. x?=w1607:bool)
            n1477 = local read "EVENT LOG"() -> (w1611:string)
            n1478 = local write "Temperature Off Command"(w1607) -> ()
            n1479 = call "Event Log.vi"("Content"="Heater Off", "EVENT LOG"=w1611) -> ("EVENT LOG"=w1610:string)  [unwired: 8 in, 1 out]
            n1480 = local write "EVENT LOG"(w1610) -> ()
          }
        }
      }
      frame True {
        n1481 = local write "Temperature Off Command"(TRUE ("Temperature Off Command")) -> ()
        n1482 = case shown="True" "Temperature On Command" {
          selector: "Temperature On Command" -> [_ w1615]
          frame False {
          }
          frame True {
            n1483 = Not(x=w1615) -> (.not. x?=w1614:bool)
            n1484 = local write "Temperature On Command"(w1614) -> ()
            n1485 = disable-structure shown="Enabled" {
